vi "Build Tree Data Type.vi"(4 "Show IDs (True)":bool=TRUE, 6 "Indent":i32, 7 "Tag Blacklist":i8[](array[numeric]), 8 "error in (no error)":errorcluster, 9 "Items":T1(array[cluster]), 10 "Child IDs":string[](array[string]), 11 "Linked List in":refnum<class "Linked List.lvclass">) -> (0 "error out":errorcluster, 1 "Items Out":T1(array[cluster]), 3 "Linked List out":refnum<class "Linked List.lvclass">)   [LabVIEW 2020, in "Linked Lists.lvlib" / "Linked List.lvclass"]
uses:
  <vilib>/gpm_packages/@cs/linked-list/Source/Linked List/Linked List/Linked List.lvclass
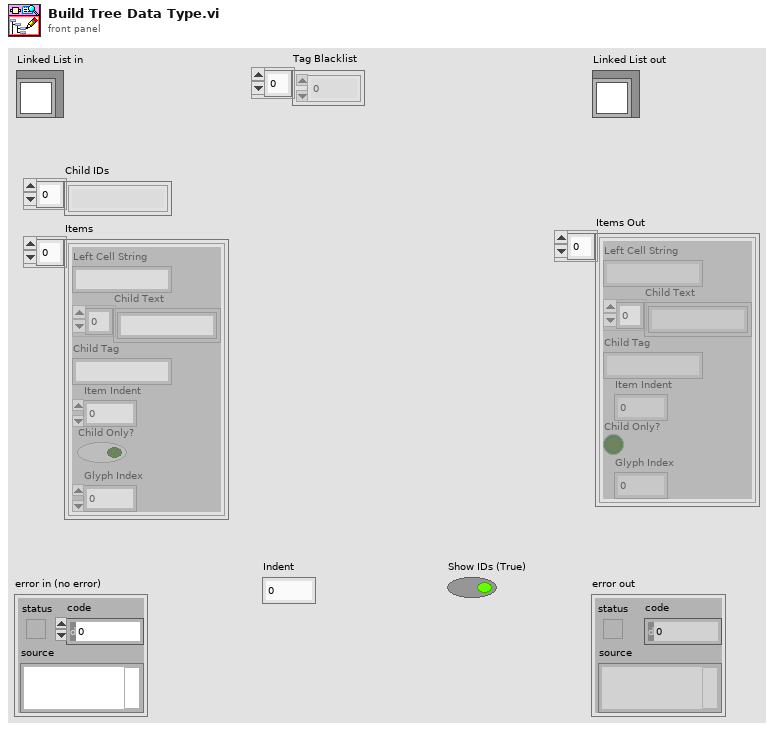
[diagram p1: front panel]
types:
  T1 = cluster{"Left Cell String":string, "Child Text":string[], "Child Tag":string, "Item Indent":i32, "Child Only?":bool, "Glyph Index":i32}[]
  T2 = cluster{"Left Cell String":string, "Child Text":string[], "Child Tag":string, "Item Indent":i32, "Child Only?":bool, "Glyph Index":i32}
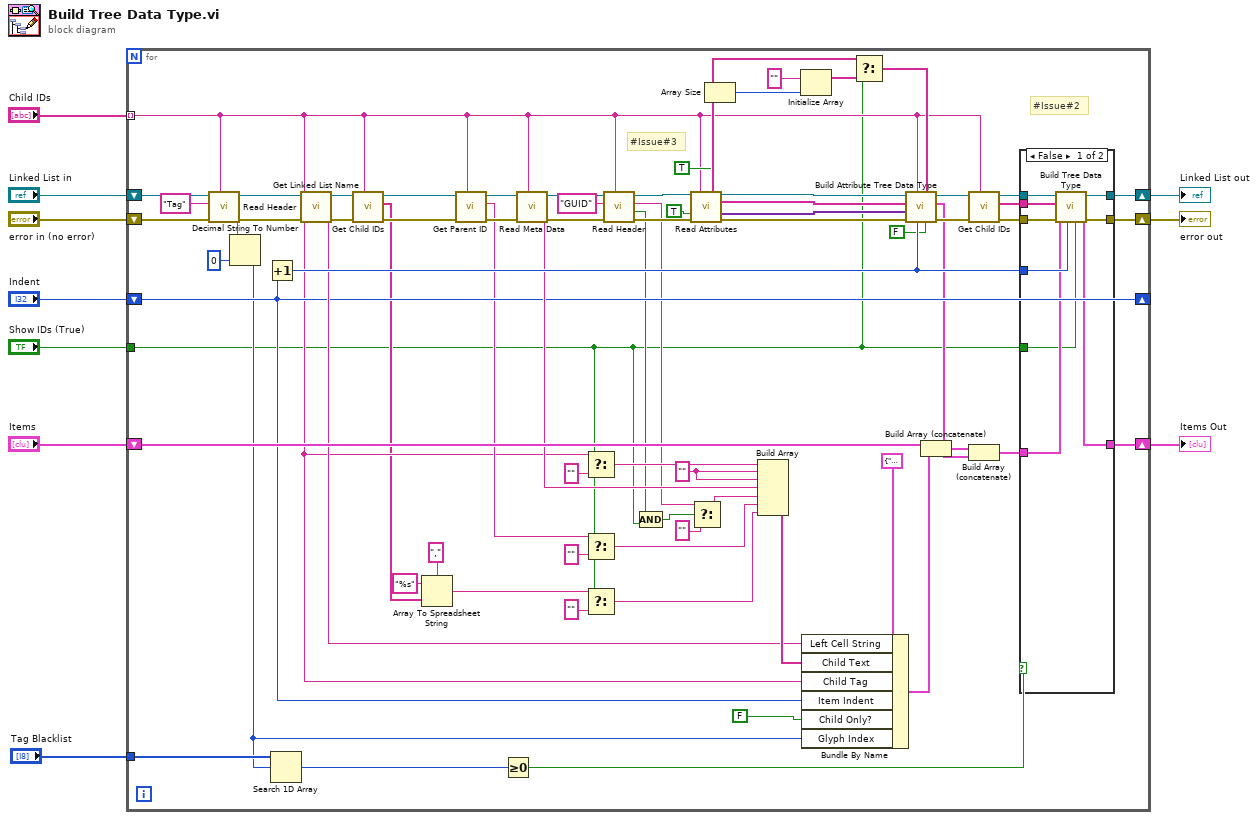
[diagram p0: block diagram]
diagram:
  n1 = for {
    shift-right: [w71] -> w9
    shift-left: "Linked List in" -> [w83]
    shift-right: [w72] -> w7
    shift-left: "error in (no error)" -> [w82]
    shift-right: [w49] -> _
    shift-left: "Indent" -> [w49]
    shift-right: [w48] -> w2
    shift-left: "Items" -> [w52]
    tunnel: "Show IDs (True)" -> [w13]
    tunnel: "Child IDs" -> [w19] mode=indexing
    tunnel: "Tag Blacklist" -> [w31]
    w39 = "" ("element")
    # "#Issue#3"
    # "#Issue#2"
    n2 = call-dynamic "Read Header.vi"("Linked List ID"=w19, "error in (no error)"=w82, "Header Name"="Tag", "Linked List in"=w83) -> ("error out"=w77:errorcluster, "Header Value"=w79:string, "Linked List out"=w78:refnum<class "Linked List.lvclass">)  [unwired: 4 in, 1 out]
    n3 = Decimal String To Number(string=w79, default (0L)=i8 0 ("default (0 I32)")) -> (number=w30:i8)  [unwired: 1 in, 1 out]
    n4 = Increment(x=w49) -> (x+1=w65:i32)
    n5 = Search 1D Array(1D array=w31, element=w30) -> (index of element=w29:i32)  [unwired: 1 in]
    n6 = call-dynamic "Get Linked List Name.vi"("error in (no error)"=w77, "Unique ID"=w19, "Linked List in"=w78) -> ("error out"=w21:errorcluster, "Linked List Name"=w51:string, "Linked List out"=w23:refnum<class "Linked List.lvclass">)  [unwired: 5 in, 1 out]
    n7 = call-dynamic "Get Child IDs.vi"("Linked List ID"=w19, "error in (no error)"=w21, "Linked List in"=w23) -> ("error out"=w20:errorcluster, "Child IDs"=w18:string[], "Linked List out"=w22:refnum<class "Linked List.lvclass">)  [unwired: 6 in]
    n8 = Array To Spreadsheet String(delimiter (Tab)=",", array=w18, 3:"%s" ("format string")) -> (spreadsheet string=w12:string)
    n9 = call-dynamic "Get Parent ID.vi"("Linked List ID"=w19, "error in (no error)"=w20, "Linked List in"=w22) -> ("error out"=w26:errorcluster, "Parent ID"=w25:string, "Linked List out"=w27:refnum<class "Linked List.lvclass">)  [unwired: 5 in, 1 out]
    n10 = Greater Or Equal To 0?(x=w29) -> (x >= 0?=w28:bool)
    n11 = call-dynamic "Read Meta Data.vi"("Linked List ID"=w19, "error in (no error)"=w26, "Linked List in"=w27) -> ("error out"=w42:errorcluster, "Meta Data"=w50:string, "Linked List out"=w44:refnum<class "Linked List.lvclass">)  [unwired: 5 in, 1 out]
    n12 = Select(t=w19, s=w13, f="") -> (s? t:f=w54:string)
    n13 = Select(t=w25, s=w13, f="") -> (s? t:f=w15:string)
    n14 = Select(t=w12, s=w13, f="") -> (s? t:f=w11:string)
    n15 = call-dynamic "Read Header.vi"("Linked List ID"=w19, "error in (no error)"=w42, "Header Name"="GUID", "Linked List in"=w44) -> ("error out"=w41:errorcluster, "found"=w37:bool, "Header Value"=w38:string, "Linked List out"=w43:refnum<class "Linked List.lvclass">)  [unwired: 4 in]
    n16 = Compound Arithmetic op=AND(w37, w13) -> (w36:bool)
    n17 = call-dynamic "Read Attributes.vi"("Linked List in"=w43, "Linked List ID"=w19, "Include Private?"=TRUE, "Flatten Pointer?"=TRUE, "error in (no error)"=w41) -> ("Linked List out"=w70:refnum<class "Linked List.lvclass">, "Attribute Names out"=w68:string[], "Attributes"=w67:variant[], "Data IDs"=w73:string[], "error out"=w69:errorcluster)  [unwired: 4 in, 2 out]
    n18 = Select(t=w38, s=w36, f="") -> (s? t:f=w35:string)
    n19 = Array Size(array=w73) -> (size(s)=w76:i32)
    n20 = Build Array(w54, w39, w39, w50, w35, w15, w11) -> (w56:string[])
    n21 = Initialize Array("" ("Name"), w76) -> (w74:string[])
    n22 = Bundle By Name(cluster=T2 {"Left Cell String"="", "Child Text"=[], "Child Tag"="", "Item Indent"=0, "Child Only?"=FALSE, "Glyph Index"=0} ("Item"), "Left Cell String"=w51, "Child Text"=w56, "Child Tag"=w19, "Item Indent"=w49, "Child Only?"=FALSE, "Glyph Index"=w30) -> (w58:T2)
    n23 = Select(t=w73, s=w13, f=w74) -> (s? t:f=w66:string[])
    n24 = call <vilib>:"Build Attribute Tree Data Type.vi"("Show Private?"=FALSE, "Attribute IDs"=w66, "Item Indent"=w65, "Linked List ID"=w19, "error in (no error)"=w69, "Attribute Values"=w67, "Attribute Names"=w68, "Linked List in"=w70) -> ("error out"=w62:errorcluster, "Tree Data Type"=w47:T1, "Linked List out"=w64:refnum<class "Linked List.lvclass">)  [unwired: 1 in]
    n25 = Build Array (concatenate)(w52, w58) -> (w57:T1)
    n26 = call-dynamic "Get Child IDs.vi"("Linked List ID"=w19, "error in (no error)"=w62, "Linked List in"=w64) -> ("error out"=w61:errorcluster, "Child IDs"=w60:string[], "Linked List out"=w63:refnum<class "Linked List.lvclass">)  [unwired: 6 in]
    n27 = Build Array (concatenate)(w57, w47) -> (w46:T1)
    n28 = case shown="False" w28 {
      tunnel: [w92 w94] -> w72
      tunnel: [w91 w95] -> w71
      tunnel: w65 -> [w90 _]
      tunnel: w63 -> [w89 w95]
      tunnel: w61 -> [w88 w94]
      tunnel: w60 -> [w87 _]
      tunnel: [w86 w93] -> w48
      tunnel: w46 -> [w85 w93]
      tunnel: w13 -> [w84 _]
      frame False {
        n29 = call-dynamic "Build Tree Data Type.vi"("Show IDs (True)"=w84, "Indent"=w90, "error in (no error)"=w88, "Items"=w85, "Child IDs"=w87, "Linked List in"=w89) -> ("error out"=w92:errorcluster, "Items Out"=w86:T1, "Linked List out"=w91:refnum<class "Linked List.lvclass">)  [unwired: 3 in]
      }
      frame True {
      }
    }
  }
  "error out" <- w7
  "Linked List out" <- w9
  "Items Out" <- w2
